vi "Verify Stored Template Path.vi"(11 "Proposed Template Path":path) -> (3 "Valid Template Path?":bool)   [LabVIEW 2016]
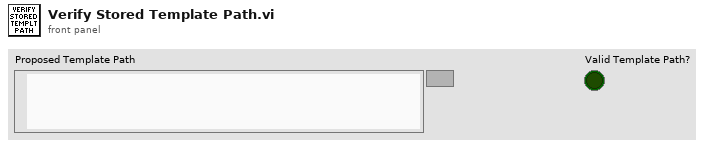
[diagram p1: front panel]
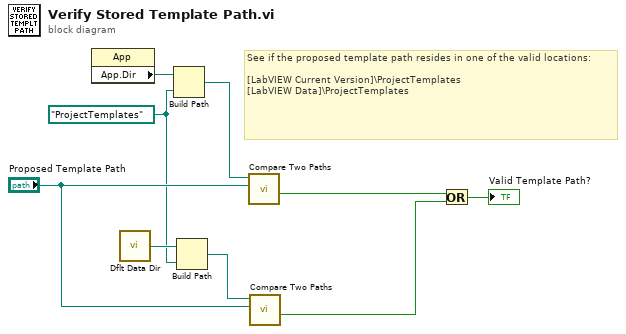
[diagram p0: block diagram]
diagram:
  w5 = path "ProjectTemplates"
  # "See if the proposed template path resides in one of the valid locations:\n\n[LabVIEW Current Version]\\ProjectTemplates\n[LabVIEW Data]\\ProjectTemplates"
  n1 = property class="App"() -> ("App.Dir"=w8:path)  [unwired: 2 in, 2 out]
  n2 = call <vilib>:"Dflt Data Dir.vi"() -> ("App:Default Data Directory"=w6:path)
  n3 = Build Path(base path=w8, name or relative path=w5) -> (appended path=w7:path)
  n4 = Build Path(base path=w6, name or relative path=w5) -> (appended path=w4:path)
  n5 = call <vilib>:"Compare Two Paths.vi"("Path 2"="Proposed Template Path", "Path 1"=w7) -> ("Path 2 Relative to Path 1?"=w3:bool)  [unwired: 6 in, 3 out]
  n6 = call <vilib>:"Compare Two Paths.vi"("Path 2"="Proposed Template Path", "Path 1"=w4) -> ("Path 2 Relative to Path 1?"=w2:bool)  [unwired: 6 in, 3 out]
  n7 = Or(x=w3, y=w2) -> (x .or. y?=→"Valid Template Path?":bool)
